vi "Steam Stats.vi"(2 "Divisor":dbl, 3 "Flow":i64) -> (0 "Pressure (bar)":dbl, 1 "Flow (kg/s)":dbl)   [LabVIEW 2023]
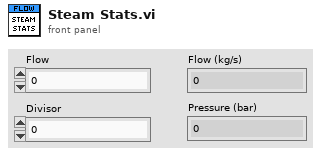
[diagram p1: front panel]
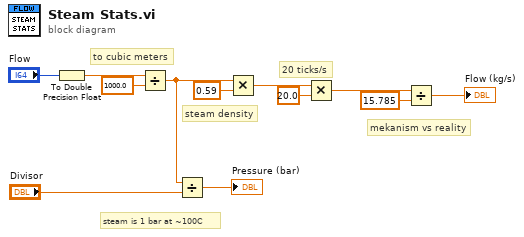
[diagram p0: block diagram]
diagram:
  # "steam is 1 bar at ~100C"
  # "mekanism vs reality"
  # "20 ticks/s"
  # "steam density"
  # "to cubic meters"
  n1 = To Double Precision Float(number="Flow") -> (double precision float=w8:dbl)
  n2 = Divide(x=w8, y=1000.0) -> (x/y=w2:dbl)
  n3 = Divide(x=w2, y="Divisor") -> (x/y=→"Pressure (bar)":dbl)
  n4 = Multiply(x=w2, y=0.59) -> (x*y=w11:dbl)
  n5 = Multiply(x=w11, y=20.0) -> (x*y=w12:dbl)
  n6 = Divide(x=w12, y=15.785) -> (x/y=→"Flow (kg/s)":dbl)
